vi "Combine_Full_Report.vi"(7 "Generate Report":bool, 8 "error in (no error)":errorcluster, 10 "XY Graph":cluster{"X":dbl, "Y":dbl}[](graph), 11 "Report Array Header":string[](array[string])) -> (0 "error out":errorcluster, 3 "Temporary test data":dbl[][](array[numeric]))   [LabVIEW 2020]
uses:
  <vilib>/Utility/NIReport.llb/Report Type.ctl
  <vilib>/Utility/file.llb/Read Delimited Spreadsheet (DBL).vi
  <vilib>/Utility/NIReport.llb/NI_report.lvclass
  <vilib>/Utility/NIReport.llb/NI_ReportGenerationCore.lvlib
  <vilib>/Utility/NIReport.llb/Excel/NI_Excel.lvclass
panel:
  out "Test Fixture (Index : 6)":string
  out "SheetName":string
  out "Target Test Signal Level":string
  out "Test Type SHORTCUT":string
  out "Measured Test Signal Level":string
  out "REQUEST NUMBER ONLY":string
  out "Test Comment (Index : 12)":string
  out "Lot/Date Code (Index : 11)":string
  out "Lot Number (Index : 10)":string
  out "Capacitance Units (Index : 9)":string
  out "Full Test Signal Level (Index : 8)":string
  out "Test Frequency (Index : 7)":string
  out "Test System (Index : 5)":string
  out "Test Type (Index : 4)":string
  out "Part Number (Index : 3)":string
  out "Date (Index : 2)":string
  out "Request Number (Index : 1)":string
  out "Operator (Index : 0)":string
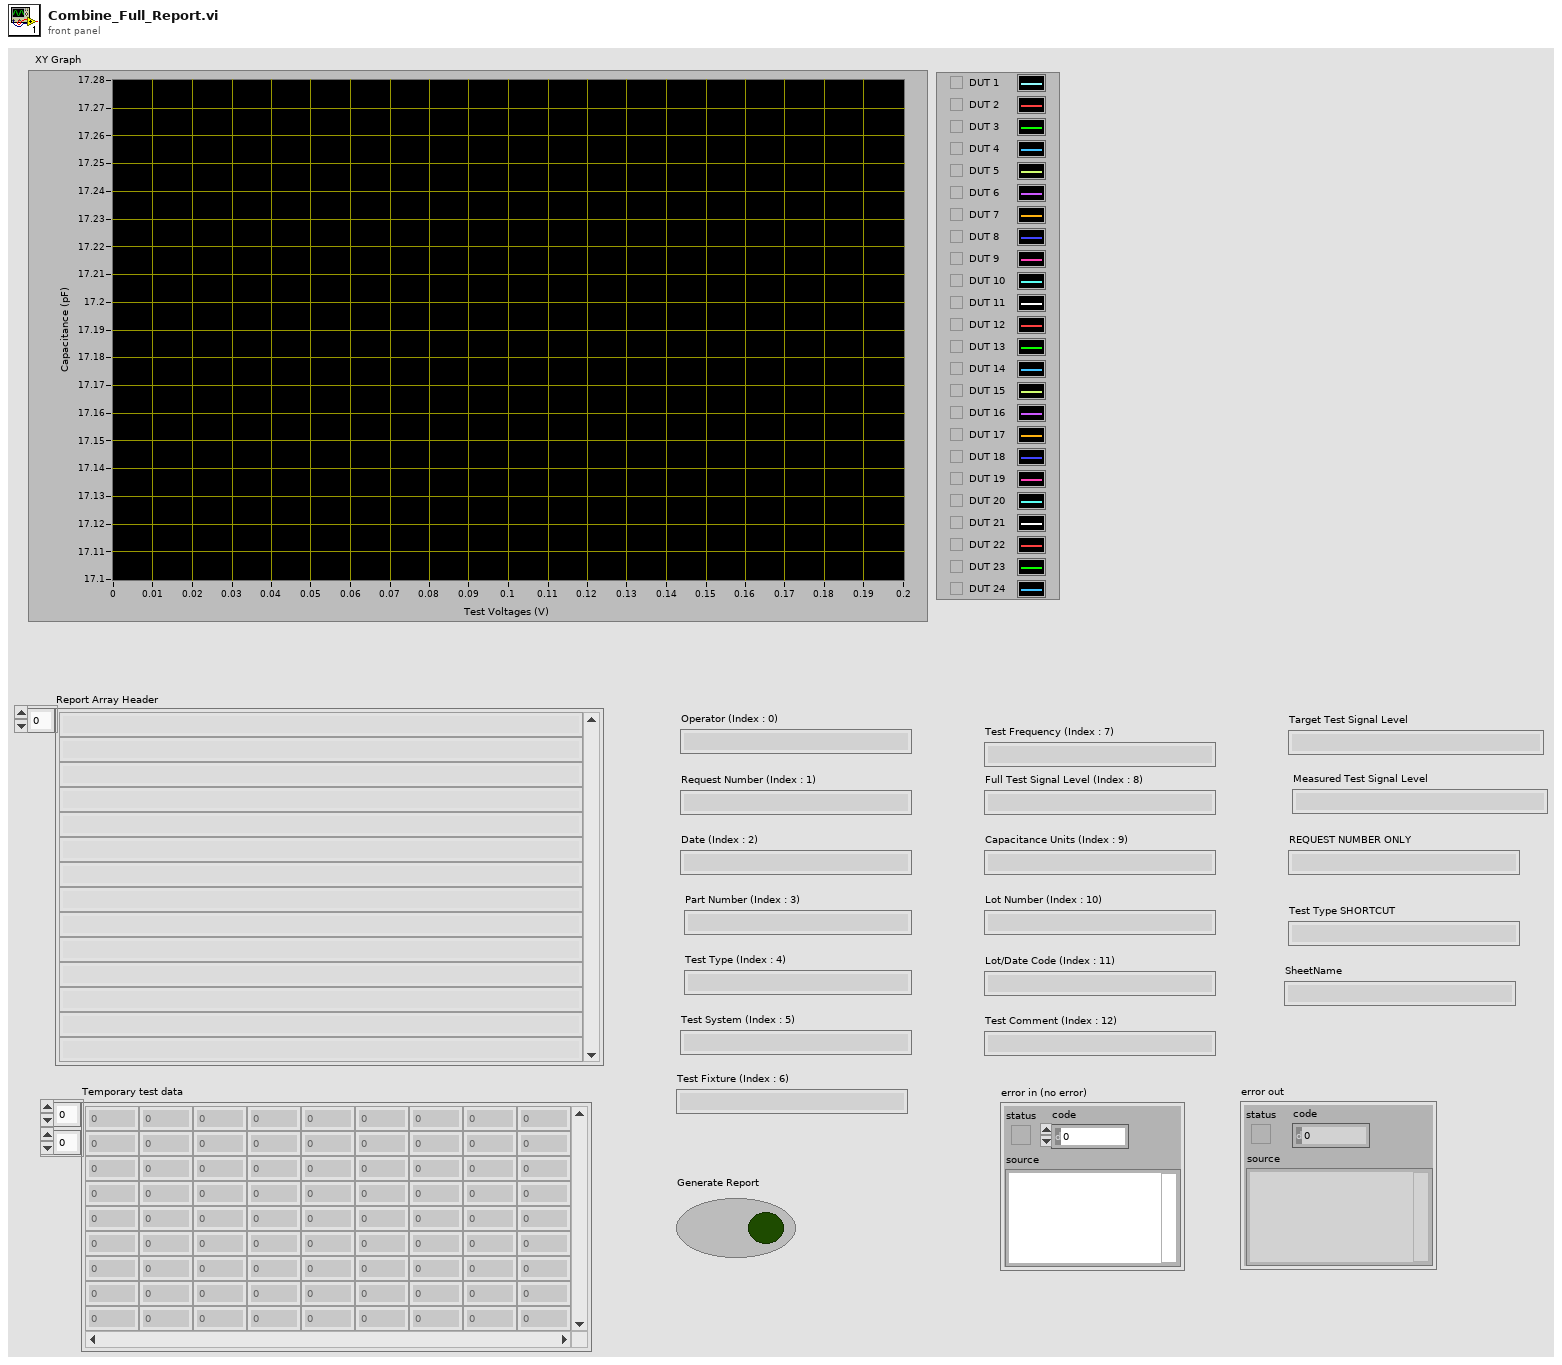
[diagram p1: front panel]
types:
  T1 = enum16{"maximized", "minimized", "normal", "no change"}
  T2 = typedef "NI_ReportGenerationCore.lvlib/Report Type.ctl" = enum16{"HTML", "Word", "Excel"}
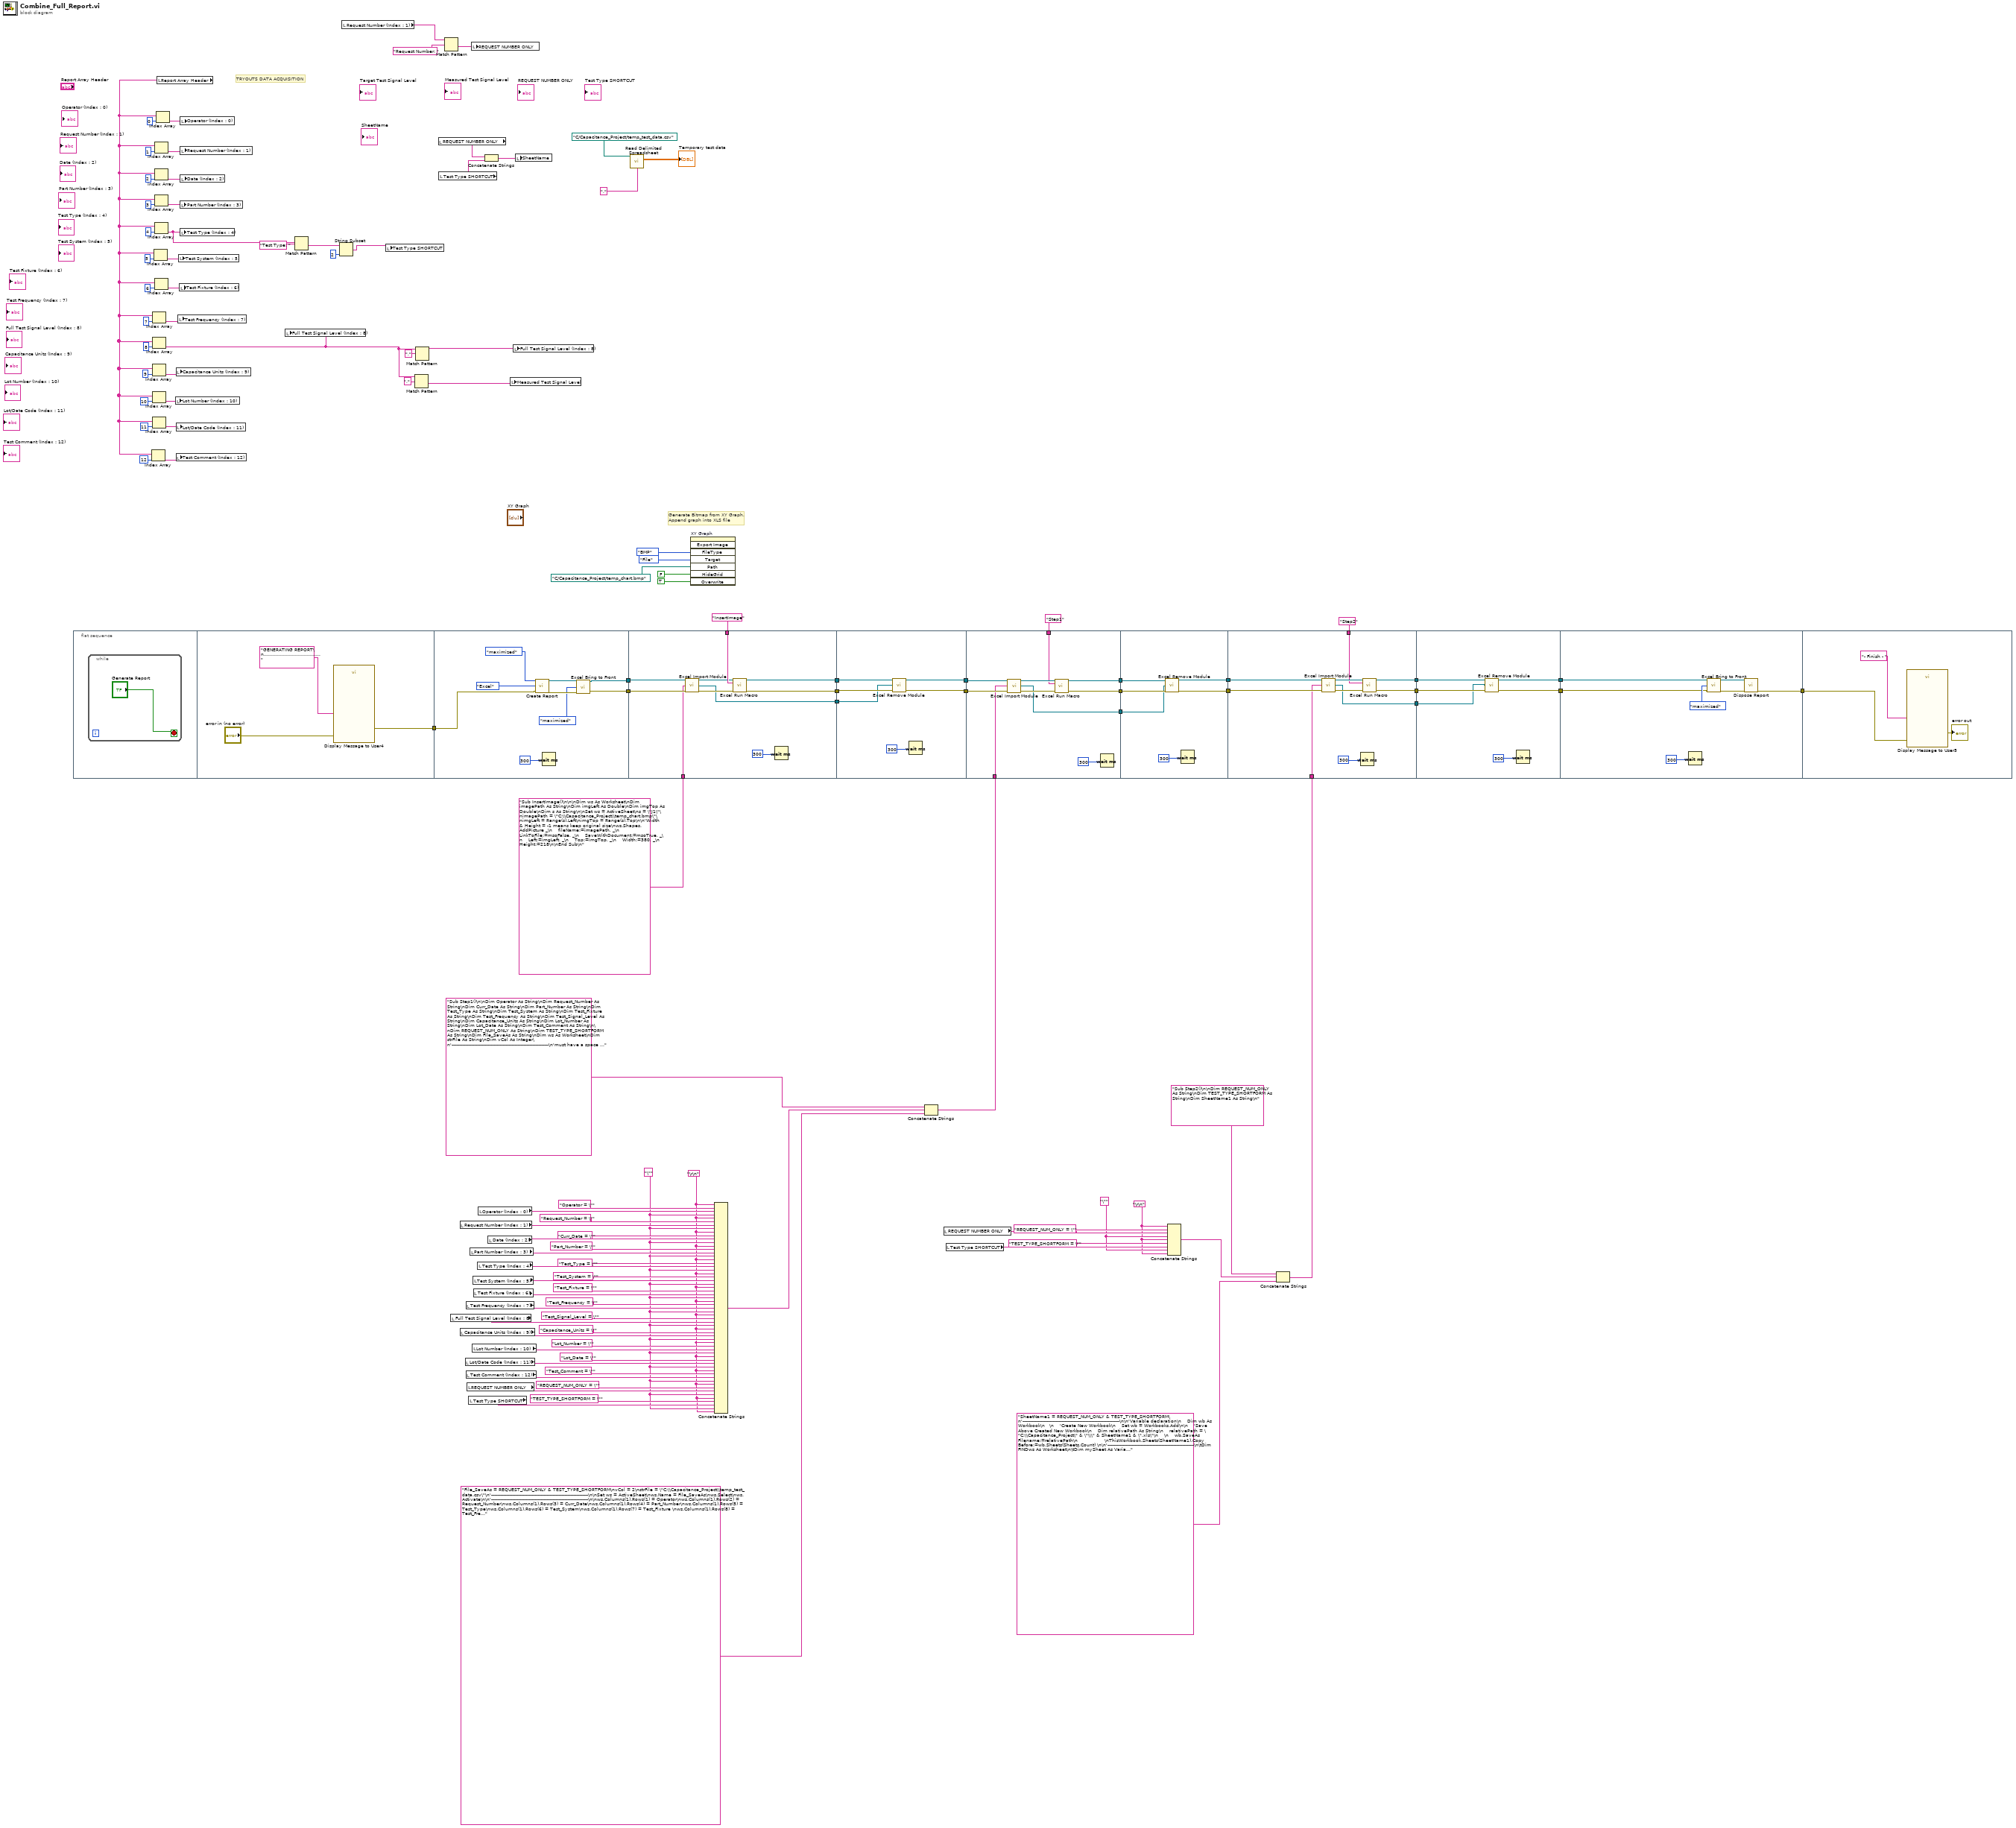
[diagram p0: block diagram]
diagram:
  w45 = "\""
  w44 = "\r\n"
  w7 = "\""
  w6 = "\r\n"
  # "Generate Bitmap from XY Graph,\nAppend graph into XLS file"
  # "TRYOUTS DATA ACQUISITION"
  n1 = flat-sequence {
    tunnel: [w120] -> w118
    tunnel: w118 -> [w125]
    tunnel: [w124] -> w35
    tunnel: [w123] -> w33
    tunnel: w35 -> [w139]
    tunnel: [w135] -> w34
    tunnel: w33 -> [w138]
    tunnel: [w134] -> w32
    tunnel: "InsertImage" ("macro name") -> [w140]
    tunnel: [w133] -> w30
    tunnel: "Sub InsertImage()\n\n\nDim ws As Worksheet\nDim imagePath As String\nDim imgLeft As Double\nDim imgTop As Double\nDim s As String\n\nSet ws = ActiveSheet\ns = \"J1\"\nimagePath = \"C:\\Capacitance_Project\\temp_chart.bmp\"\nimgLeft = Range(s).Left\nimgTop = Range(s).Top\n\n'Width & Height = -1 means keep original size\nws.Shapes.AddPicture _\n    fileName:=imagePath, _\n    LinkToFile:=msoFalse, _\n    SaveWithDocument:=msoTrue, _\n    Left:=imgLeft, _\n    Top:=imgTop, _\n    Width:=380, _\n    Height:=218\n\nEnd Sub\n" ("module code (\"\")") -> [w132]
    tunnel: w34 -> [w146]
    tunnel: [w144] -> w37
    tunnel: w32 -> [w145]
    tunnel: [w143] -> w36
    tunnel: w30 -> [w142]
    tunnel: w37 -> [w155]
    tunnel: w36 -> [w154]
    tunnel: [w153] -> w117
    tunnel: [w152] -> w116
    tunnel: [w151] -> w115
    tunnel: w65 -> [w150]
    tunnel: "Step1" ("macro name") -> [w149]
    tunnel: w117 -> [w163]
    tunnel: w116 -> [w162]
    tunnel: [w161] -> w61
    tunnel: [w160] -> w60
    tunnel: w115 -> [w159]
    tunnel: w61 -> [w168]
    tunnel: [w167] -> w59
    tunnel: w60 -> [w169]
    tunnel: [w170] -> w57
    tunnel: "Step2" ("macro name") -> [w166]
    tunnel: [w165] -> w54
    tunnel: w53 -> [w164]
    tunnel: w59 -> [w176]
    tunnel: [w175] -> w58
    tunnel: w57 -> [w178]
    tunnel: [w177] -> w56
    tunnel: w54 -> [w174]
    tunnel: w58 -> [w181]
    tunnel: w56 -> [w180]
    tunnel: [w183] -> w114
    tunnel: w114 -> [w188]
    frame #0 {
      n2 = while {
        stop <- "Generate Report" stop-if-true
      }
    }
    frame #1 {
      n3 = call "Display Message to User4"("error in (no error)"="error in (no error)", "Message"="GENERATING REPORT\n......................................") -> ("error out"=w120:errorcluster)  [unwired: 8 in, 1 out]
    }
    frame #2 {
      n4 = call <vilib>:"Create Report.vi"("window state (normal)"=T1."maximized", "report type"=Report_Type."Excel", "error in (no error)"=w125) -> ("report out"=w128:refnum<class "NI_report.lvclass">, "error out"=w129:errorcluster)  [unwired: 11 in]
      n5 = Wait (ms)(milliseconds to wait=u32 300 ("millisecond timer value")) -> ()  [unwired: 1 out]
      n6 = call <vilib>:"Excel Bring to Front.vi"("report in"=w128, "window state (maximized)"=enum16{"maximized", "minimized", "normal"}."maximized", "error in (no error)"=w129) -> ("report out"=w124:refnum<class "NI_report.lvclass">, "error out"=w123:errorcluster)  [unwired: 11 in]
    }
    frame #3 {
      n7 = call <vilib>:"Excel Import Module.vi"("report in"=w139, "module code (\"\")"=w132, "error in (no error)"=w138) -> ("report out"=w136:refnum<class "NI_report.lvclass">, "module reference"=w133:refnum<k7>, "error out"=w137:errorcluster)  [unwired: 10 in]
      n8 = call <vilib>:"Excel Run Macro.vi"("report in"=w136, "macro name"=w140, "error in (no error)"=w137) -> ("report out"=w135:refnum<class "NI_report.lvclass">, "error out"=w134:errorcluster)  [unwired: 10 in, 1 out]
      n9 = Wait (ms)(milliseconds to wait=u32 300 ("millisecond timer value")) -> ()  [unwired: 1 out]
    }
    frame #4 {
      n10 = call <vilib>:"Excel Remove Module.vi"("report in"=w146, "module reference"=w142, "error in (no error)"=w145) -> ("report out"=w144:refnum<class "NI_report.lvclass">, "error out"=w143:errorcluster)  [unwired: 11 in]
      n11 = Wait (ms)(milliseconds to wait=u32 300 ("millisecond timer value")) -> ()  [unwired: 1 out]
    }
    frame #5 {
      n12 = call <vilib>:"Excel Import Module.vi"("report in"=w155, "module code (\"\")"=w150, "error in (no error)"=w154) -> ("report out"=w157:refnum<class "NI_report.lvclass">, "module reference"=w151:refnum<k7>, "error out"=w156:errorcluster)  [unwired: 10 in]
      n13 = call <vilib>:"Excel Run Macro.vi"("report in"=w157, "macro name"=w149, "error in (no error)"=w156) -> ("report out"=w153:refnum<class "NI_report.lvclass">, "error out"=w152:errorcluster)  [unwired: 10 in, 1 out]
      n14 = Wait (ms)(milliseconds to wait=u32 300 ("millisecond timer value")) -> ()  [unwired: 1 out]
    }
    frame #6 {
      n15 = call <vilib>:"Excel Remove Module.vi"("report in"=w163, "module reference"=w159, "error in (no error)"=w162) -> ("report out"=w161:refnum<class "NI_report.lvclass">, "error out"=w160:errorcluster)  [unwired: 11 in]
      n16 = Wait (ms)(milliseconds to wait=u32 300 ("millisecond timer value")) -> ()  [unwired: 1 out]
    }
    frame #7 {
      n17 = call <vilib>:"Excel Import Module.vi"("report in"=w168, "module code (\"\")"=w164, "error in (no error)"=w169) -> ("report out"=w171:refnum<class "NI_report.lvclass">, "module reference"=w165:refnum<k7>, "error out"=w172:errorcluster)  [unwired: 10 in]
      n18 = Wait (ms)(milliseconds to wait=u32 300 ("millisecond timer value")) -> ()  [unwired: 1 out]
      n19 = call <vilib>:"Excel Run Macro.vi"("report in"=w171, "macro name"=w166, "error in (no error)"=w172) -> ("report out"=w167:refnum<class "NI_report.lvclass">, "error out"=w170:errorcluster)  [unwired: 10 in, 1 out]
    }
    frame #8 {
      n20 = call <vilib>:"Excel Remove Module.vi"("report in"=w176, "module reference"=w174, "error in (no error)"=w178) -> ("report out"=w175:refnum<class "NI_report.lvclass">, "error out"=w177:errorcluster)  [unwired: 11 in]
      n21 = Wait (ms)(milliseconds to wait=u32 300 ("millisecond timer value")) -> ()  [unwired: 1 out]
    }
    frame #9 {
      n22 = Wait (ms)(milliseconds to wait=u32 300 ("millisecond timer value")) -> ()  [unwired: 1 out]
      n23 = call <vilib>:"Excel Bring to Front.vi"("report in"=w181, "window state (maximized)"=enum16{"maximized", "minimized", "normal"}."maximized", "error in (no error)"=w180) -> ("report out"=w185:refnum<class "NI_report.lvclass">, "error out"=w184:errorcluster)  [unwired: 11 in]
      n24 = call-dynamic "Dispose Report.vi"("report in"=w185, "error in (no error)"=w184) -> ("error out"=w183:errorcluster)  [unwired: 13 in]
    }
    frame #10 {
      n25 = call "Display Message to User5"("error in (no error)"=w188, "Message"="- Finish - ") -> ("error out"=→"error out":errorcluster)  [unwired: 8 in, 1 out]
    }
  }
  n26 = local read "Report Array Header"() -> (w26:string[])
  n27 = Index Array(array=w26, index=12) -> (element=w83:string)
  n28 = Index Array(array=w26, index=9) -> (element=w86:string)
  n29 = Index Array(array=w26, index=10) -> (element=w85:string)
  n30 = Index Array(array=w26, index=11) -> (element=w84:string)
  n31 = Index Array(array=w26, index=7) -> (element=w87:string)
  n32 = Index Array(array=w26, index=8) -> (element=w62:string)
  n33 = Index Array(array=w26, index=5) -> (element=w88:string)
  n34 = Index Array(array=w26, index=6) -> (element=w28:string)
  n35 = Index Array(array=w26, index=1) -> (element=w92:string)
  n36 = Index Array(array=w26, index=2) -> (element=w91:string)
  n37 = Index Array(array=w26, index=3) -> (element=w90:string)
  n38 = Index Array(array=w26, index=4) -> (element=w89:string)
  n39 = Index Array(array=w26, index=0) -> (element=w93:string)
  n40 = local write "Lot Number (Index : 10)"(w85) -> ()
  n41 = local write "Capacitance Units (Index : 9)"(w86) -> ()
  n42 = local write "Lot/Date Code (Index : 11)"(w84) -> ()
  n43 = local write "Test Comment (Index : 12)"(w83) -> ()
  n44 = local write "Test Frequency (Index : 7)"(w87) -> ()
  n45 = local write "Test System (Index : 5)"(w88) -> ()
  n46 = local write "Test Fixture (Index : 6)"(w28) -> ()
  n47 = local write "Part Number (Index : 3)"(w90) -> ()
  n48 = local write "Test Type (Index : 4)"(w89) -> ()
  n49 = local write "Operator (Index : 0)"(w93) -> ()
  n50 = local write "Request Number (Index : 1)"(w92) -> ()
  n51 = local write "Date (Index : 2)"(w91) -> ()
  n52 = local write "Full Test Signal Level (Index : 8)"(w62) -> ()
  n53 = Match Pattern(string=w89, regular expression="Test Type: ") -> (after substring=w43:string)  [unwired: 1 in, 3 out]
  n54 = String Subset(string=w43, length (rest)=2 ("length (rest)")) -> (substring=w42:string)  [unwired: 1 in]
  n55 = local read "Request Number (Index : 1)"() -> (w113:string)
  n56 = local write "Test Type SHORTCUT"(w42) -> ()
  n57 = Match Pattern(string=w62, regular expression=",") -> (after substring=w95:string)  [unwired: 1 in, 3 out]
  n58 = Match Pattern(string=w62, regular expression=",") -> (before substring=w98:string)  [unwired: 1 in, 3 out]
  n59 = local read "REQUEST NUMBER ONLY"() -> (w40:string)
  n60 = local read "Test Type SHORTCUT"() -> (w39:string)
  n61 = Match Pattern(string=w113, regular expression="Request Number: ") -> (after substring=w97:string)  [unwired: 1 in, 3 out]
  n62 = local read "Full Test Signal Level (Index : 8)"() -> (w20:string)
  n63 = local read "Request Number (Index : 1)"() -> (w75:string)
  n64 = local read "Capacitance Units (Index : 9)"() -> (w18:string)
  n65 = local read "Lot/Date Code (Index : 11)"() -> (w14:string)
  n66 = local read "Test Frequency (Index : 7)"() -> (w22:string)
  n67 = local read "Test Comment (Index : 12)"() -> (w12:string)
  n68 = local read "REQUEST NUMBER ONLY"() -> (w10:string)
  n69 = local read "Test Type SHORTCUT"() -> (w8:string)
  n70 = local read "Part Number (Index : 3)"() -> (w71:string)
  n71 = local write "REQUEST NUMBER ONLY"(w97) -> ()
  n72 = local read "Lot Number (Index : 10)"() -> (w16:string)
  n73 = local read "Test System (Index : 5)"() -> (w63:string)
  n74 = local read "Test Fixture (Index : 6)"() -> (w24:string)
  n75 = local read "Test Type (Index : 4)"() -> (w69:string)
  n76 = local read "Operator (Index : 0)"() -> (w77:string)
  n77 = Concatenate Strings(w40, w39) -> (w38:string)
  n78 = local read "Date (Index : 2)"() -> (w73:string)
  n79 = local write "Measured Test Signal Level"(w95) -> ()
  n80 = local write "Full Test Signal Level (Index : 8)"(w98) -> ()
  n81 = local write "SheetName"(w38) -> ()
  n82 = call-poly <vilib>:"Read Delimited Spreadsheet.vi"("file path (dialog if empty)"=path "C:/Capacitance_Project/temp_test_data.csv", "delimiter (\\t)"="," ("delimiter (\\t)")) -> ("all rows"=→"Temporary test data":dbl[][])  [unwired: 8 in, 5 out]
  n83 = invoke on="XY Graph" class="XYGraph (strict)" method="Export Image"("FileType"=enum32{"BMP", "EPS", "EMF", "PICT"}."BMP" ("File Type"), "Target"=enum32{"File", "Clipboard"}."File", "Path"=path "C:/Capacitance_Project/temp_chart.bmp", "HideGrid"=FALSE ("Hide Grid"), "Overwrite"=TRUE ("Always Overwrite")) -> ()  [unwired: 3 in, 8 out]
  n84 = Concatenate Strings(w6, "Operator = \"", w77, w7, w6, "Request_Number = \"" ("string"), w75, w7, w6, "Curr_Date = \"" ("string"), w73, w7, w6, "Part_Number = \"" ("string"), w71, w7, w6, "Test_Type = \"" ("string"), w69, w7, w6, "Test_System = \"" ("string"), w63, w7, w6, "Test_Fixture = \"", w24, w7, w6, "Test_Frequency = \"" ("string"), w22, w7, w6, "Test_Signal_Level = \"" ("string"), w20, w7, w6, "Capacitance_Units = \"" ("string"), w18, w7, w6, "Lot_Number = \"" ("string"), w16, w7, w6, "Lot_Date = \"" ("string"), w14, w7, w6, "Test_Comment = \"" ("string"), w12, w7, w6, "REQUEST_NUM_ONLY = \"" ("string"), w10, w7, w6, "TEST_TYPE_SHORTFORM = \"" ("string"), w8, w7, w6) -> (w67:string)
  n85 = Concatenate Strings("Sub Step1()\n\nDim Operator As String\nDim Request_Number As String\nDim Curr_Date As String\nDim Part_Number As String\nDim Test_Type As String\nDim Test_System As String\nDim Test_Fixture As String\nDim Test_Frequency As String\nDim Test_Signal_Level As String\nDim Capacitance_Units As String\nDim Lot_Number As String\nDim Lot_Date As String\nDim Test_Comment As String\n\nDim REQUEST_NUM_ONLY As String\nDim TEST_TYPE_SHORTFORM As String\nDim File_SaveAs As String\nDim ws As Worksheet\nDim strFile As String\nDim vCol As Integer\n'-----------------------------------------------------------------\n'must have a space after :_", w67, "File_SaveAs = REQUEST_NUM_ONLY & TEST_TYPE_SHORTFORM\nvCol = 2\nstrFile = \"C:\\Capacitance_Project\\temp_test_data.csv\"\n'-----------------------------------------------------------------\n\nSet ws = ActiveSheet\nws.Name = File_SaveAs\nws.Select\nws.Activate\n\n'-----------------------------------------------------------------\n\nws.Columns(1).Rows(1) = Operator\nws.Columns(1).Rows(2) = Request_Number\nws.Columns(1).Rows(3) = Curr_Date\nws.Columns(1).Rows(4) = Part_Number\nws.Columns(1).Rows(5) = Test_Type\nws.Columns(1).Rows(6) = Test_System\nws.Columns(1).Rows(7) = Test_Fixture \nws.Columns(1).Rows(8) = Test_Frequency\nws.Columns(1).Rows(9) = Test_Signal_Level\nws.Columns(1).Rows(10) = Capacitance_Units\nws.Columns(1).Rows(11) = Lot_Number\nws.Columns(1).Rows(12) = Lot_Date\nws.Columns(1).Rows(13) = Test_Comment\n\n'-----------------------------------------------------------------\n\n'-----------------------------------------------------------------\n''https://stackoverflow.com/questions/12197274/is-there-a-way-to-import-data-from-csv-to-active-excel-sheet\nWith ws.QueryTables.Add(Connection:=\"TEXT;\" & strFile, Destination:=ws.Range(\"A17\"))\n     .TextFileParseType = xlDelimited\n     .TextFileCommaDelimiter = True\n     .Refresh\nEnd With\n\nWith ws\n'https://www.extendoffice.com/documents/excel/5315-excel-restore-default-cell-size.html\n     .Cells.UseStandardHeight = True\n     .Cells.UseStandardWidth = True\n     .Columns(1).Rows(16) = \"Serial#\"\n     .Columns(1).Rows(17) = \"Voltage\"\n    \n    Do While ((.Cells(17, vCol).Value <> \"\") And (.Cells(17, vCol).Value <> \"Voltage\"))\n    .Cells(16, vCol).Value = (\"C @ \" & (.Cells(17, vCol).Value) & \" V\")\n    vCol = vCol + 1\n    Loop\n    \nEnd With\n\n\nEnd Sub" ("module code (\"\")")) -> (w65:string)
  n86 = local read "REQUEST NUMBER ONLY"() -> (w48:string)
  n87 = local read "Test Type SHORTCUT"() -> (w46:string)
  n88 = Concatenate Strings(w44, "REQUEST_NUM_ONLY = \"" ("string"), w48, w45, w44, "TEST_TYPE_SHORTFORM = \"" ("string"), w46, w45, w44) -> (w51:string)
  n89 = Concatenate Strings("Sub Step2()\n\nDim REQUEST_NUM_ONLY As String\nDim TEST_TYPE_SHORTFORM As String\nDim SheetName1 As String\n", w51, "SheetName1 = REQUEST_NUM_ONLY & TEST_TYPE_SHORTFORM\n'-----------------------------------------------------------------\n\n'Variable declaration\n    Dim wb As Workbook\n   \n    'Create New Workbook\n    Set wb = Workbooks.Add\n\n    'Save Above Created New Workbook\n    Dim relativePath As String\n    relativePath = \"C:\\Capacitance_Project\" & \"\\\" & SheetName1 & \".xls\"\n    \n    wb.SaveAs Filename:=relativePath\n                  \nThisWorkbook.Sheets(SheetName1).Copy Before:=wb.Sheets(Sheets.Count) \n\n'----------------------------------------------------------\n\tDim FINDws As Worksheet\n\tDim mySheet As Variant\n\t\n\tmySheet = SheetName1\n\nFor Each FINDws In wb.Worksheets\n    If mySheet <> FINDws.Name Then\n      FINDws.Delete\n    End If\nNext FINDws \n\nwb.Save\nwb.Close            \n\n\nEnd Sub" ("module code (\"\")")) -> (w53:string)
